vi "Reboot.vi"   [LabVIEW 2011]
panel:
  # "正在重新启动程序，请等待……"
types:
  T1 = enum32{"Invalid", "Standard", "Closed", "Hidden", "Minimized", "Maximized"}
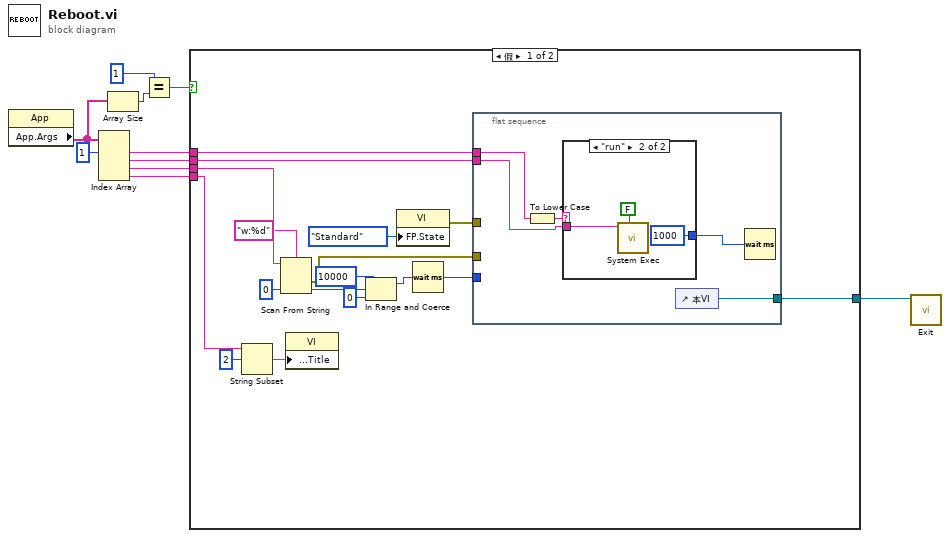
[diagram p0: block diagram]
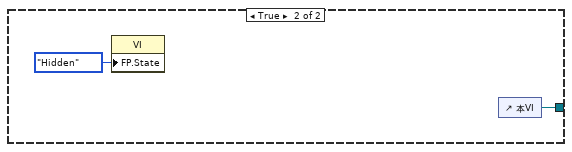
[diagram p3: hidden frame]
diagram:
  n1 = property class="App"() -> ("App.Args"=w5:string[])  [unwired: 2 in, 2 out]
  n2 = Index Array(array=w5, index #1=1 ("索引")) -> (element #1=w8:string, element #2=w7:string, element #3=w6:string, element #4=w1:string)  [unwired: 3 in]
  n3 = Array Size(array=w5) -> (size(s)=w4:i32)
  n4 = Equal?(x=1, y=w4) -> (x = y?=w2:bool)
  n5 = case shown="假" w2 {
    tunnel: [w27 w37] -> w10
    tunnel: w8 -> [w23 _]
    tunnel: w7 -> [w22 _]
    tunnel: w6 -> [w21 _]
    tunnel: w1 -> [w14 _]
    frame False {
      n6 = String Subset(string=w14, offset (0)=2 ("偏移量(0)")) -> (substring=w12:string)  [unwired: 1 in]
      n7 = Scan From String(format string="w:%d" ("格式字符串"), input string=w21, default 1=u32 0 ("等待时间（毫秒）")) -> (error out=w15:errorcluster, output 1=w19:u32)  [unwired: 2 in, 2 out]
      n8 = property class="VI"("Front Panel.Title"=w12) -> ()  [unwired: 2 in, 2 out]
      n9 = In Range and Coerce(upper limit=u32 10000 ("上限"), x=w19, lower limit=u32 0 ("下限")) -> (coerced(x)=w16:u32)  [unwired: 1 out]
      n10 = property class="VI"("FP.State"=T1."Standard" ("前面板窗口:状态")) -> (error out=w25:errorcluster)  [unwired: 2 in, 1 out]
      n11 = Wait (ms)(milliseconds to wait=w16) -> (millisecond timer value=w24:u32)
      n12 = flat-sequence {
        tunnel: [w32] -> w27
        tunnel: w25 -> [_]
        tunnel: w24 -> [_]
        tunnel: w23 -> [w30]
        tunnel: w22 -> [w29]
        tunnel: w15 -> [_]
        frame #0 {
          n13 = To Lower Case(string=w30) -> (all lower case string=w31:string)
          n14 = case shown="\"run\"" w31 {
            tunnel: w29 -> [_ w35]
            tunnel: [_ u32 1000 ("等待时间（毫秒）")] -> w28
            frame "假", Default {
            }
            frame "run" {
              n15 = call <vilib>:"System Exec.vi"("wait until completion? (T)"=FALSE, "command line"=w35) -> ()  [unwired: 6 in, 4 out]
            }
          }
          n16 = control-ref of="本VI"() -> (w32:refnum<vi>)
          n17 = Wait (ms)(milliseconds to wait=w28) -> ()  [unwired: 1 out]
        }
      }
    }
    frame True {
      n18 = property class="VI"("FP.State"=T1."Hidden" ("前面板窗口:状态")) -> ()  [unwired: 2 in, 2 out]
      n19 = control-ref of="本VI"() -> (w37:refnum<vi>)
    }
  }
  n20 = call "Exit.vi"("VI引用"=w10) -> ()  [unwired: 10 in, 1 out]
